vi "Read Trace (Reflection Measurement).vi"(8 "error in (no error)":errorcluster, 9 "Timeout (10000ms)":i32=10000, 10 "Data Type (0: Data)":i32(ring) items=["Data", "Memory"], 11 "VISA resource name":refnum<visa-resource-name>) -> (0 "error out":errorcluster, 2 "Trace Data":dbl[](array[numeric]), 3 "VISA resource name out":refnum<visa-resource-name>)   [LabVIEW 2022 SP3, in "Agilent N934X Series.lvlib"]
doc: "Reads the trace of Reflection Measurement from the spectrum analyzer.\n\nNote:\nThis VI is only applicable for N9321C, N9322C, N9323C, N9324C models."
uses:
  <instrlib>/Agilent N934X Series/Agilent N934X Series.lvlib
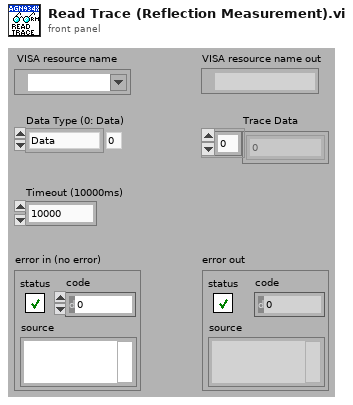
[diagram p1: front panel]
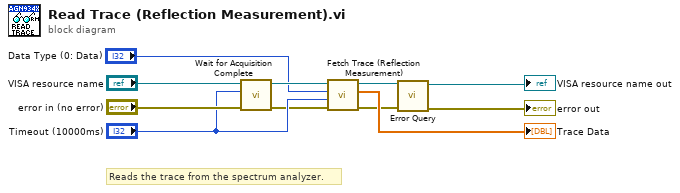
[diagram p0: block diagram]
diagram:
  # "Reads the trace from the spectrum analyzer."
  n1 = call <instrlib>:"Wait for Acquisition Complete.vi"("error in (no error)"="error in (no error)", "Maximum Time (10000 ms)"="Timeout (10000ms)", "VISA resource name"="VISA resource name") -> ("error out"=w5:errorcluster, "VISA resource name out"=w7:refnum<visa-resource-name>)  [unwired: 7 in]
  n2 = call <instrlib>:"Fetch Trace (Reflection Measurement).vi"("error in (no error)"=w5, "Timeout (10000ms)"="Timeout (10000ms)", "Data Type (0: Data)"="Data Type (0: Data)", "VISA resource name"=w7) -> ("error out"=w2:errorcluster, "Trace Data"=→"Trace Data":dbl[], "VISA resource name out"=w4:refnum<visa-resource-name>)  [unwired: 5 in]
  n3 = call <instrlib>:"Error Query.vi"("error in (no error)"=w2, "VISA resource name"=w4) -> ("error out"=→"error out":errorcluster, "VISA resource name out"=→"VISA resource name out":refnum<visa-resource-name>)  [unwired: 6 in, 2 out]
